vi "Do.vi"(8 "error in (no error)":errorcluster, 10 "Actor in":refnum<class "Actor.lvclass">, 11 "Readout Msg":refnum<class "Readout Msg.lvclass">) -> (0 "error out":errorcluster, 2 "Actor out":refnum<class "Actor.lvclass">)   [LabVIEW 2019, in "BNT_DAQmx.lvlib" / "Readout Msg.lvclass"]
doc: "This VI delivers the message to the actor by calling the appropriate method(s) on the actor."
uses:
  Readout Msg.lvclass
  BNT_DAQmx-MCSV/BNT_DAQmx-MCSV.lvclass
  CSPP_Core/Messages/CSPP_AsyncCallbackMsg/CSPP_AsyncCallback Msg.lvclass
  C:/Program Files (x86)/National Instruments/LabVIEW 2017/vi.lib/ActorFramework/Actor/Actor.lvclass
  <vilib>/ActorFramework/Actor/Actor.lvclass
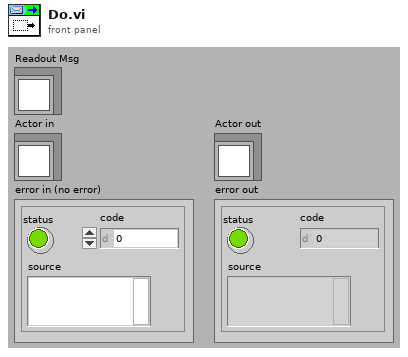
[diagram p1: front panel]
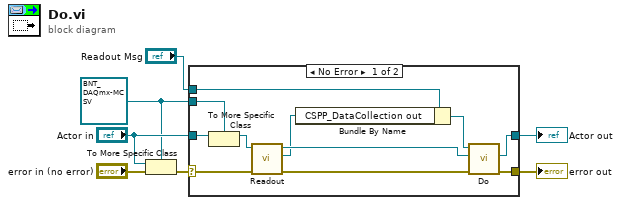
[diagram p0: block diagram]
diagram:
  w2 = refnum<class "BNT_DAQmx-MCSV.lvclass"> refnum ("Actor in")
  n1 = To More Specific Class(target class=w2, reference="Actor in", error in="error in (no error)") -> (error out=w6:errorcluster)  [unwired: 1 out]
  n2 = case shown="No Error" w6 {
    selector: w6 -> [w18 w20]
    tunnel: [w15 w20] -> w5
    tunnel: [w14 w19] -> w4
    tunnel: "Actor in" -> [w17 w19]
    tunnel: w2 -> [w16 _]
    tunnel: "Readout Msg" -> [w12 _]
    frame No Error {
      n3 = To More Specific Class ("To More Specific Class (internal)")(target class=w16, reference=w17) -> (specific class reference=w10:refnum<class "BNT_DAQmx-MCSV.lvclass">)  [unwired: 1 in, 1 out]
      n4 = call "Readout.vi"("Error In"=w18, "BNT_DAQmx-MCSV in"=w10) -> ("Error Out"=w13:errorcluster, "CSPP_DataCollection out"=w8:refnum<class "CSPP_DataCollection.lvclass">, "BNT_DAQmx-MCSV out"=w9:refnum<class "BNT_DAQmx-MCSV.lvclass">)  [unwired: 7 in]
      n5 = Bundle By Name ("Parent-Bundler")(cluster=w12, "CSPP_DataCollection out"=w8) -> (w11:refnum<class "Readout Msg.lvclass">)
      n6 = call-parent "Do.vi"("error in (no error)"=w13, "Actor in"=w9, "CSPP_AsyncCallback Msg"=w11) -> ("error out"=w15:errorcluster, "Actor out"=w14:refnum<class "Actor.lvclass">)  [unwired: 7 in]
    }
    frame Error {
    }
  }
  "error out" <- w5
  "Actor out" <- w4
